vi "Inst_K2002.vi"(8 "error in":errorcluster, 10 "All Message Queues in":T1, 11 "Prueba31 in":refnum<class "Prueba21.lvclass">) -> (0 "error out":errorcluster)   [LabVIEW 2019, in "Prueba21.lvclass"]
uses:
  Prueba21.lvclass
  QMH/Message Queue/All Message Queues.ctl
  QMH/Message Queue/Message Cluster.ctl
  Prueba21.lvclass/Prueba21.ctl
  <vilib>/Utility/error.llb/Error Cluster From Error Code.vi
  QMH/Message Queue/Enqueue Message (Single).vi
  <vilib>/ErrorRing/Error Ring.xnode
  QMH/Message Queue/Message Queue.lvlib
  Instrumento/Keithley2002/Keithley2002.lvclass
panel:
  out "All States":string[](array[string])
  out "Actual State":string
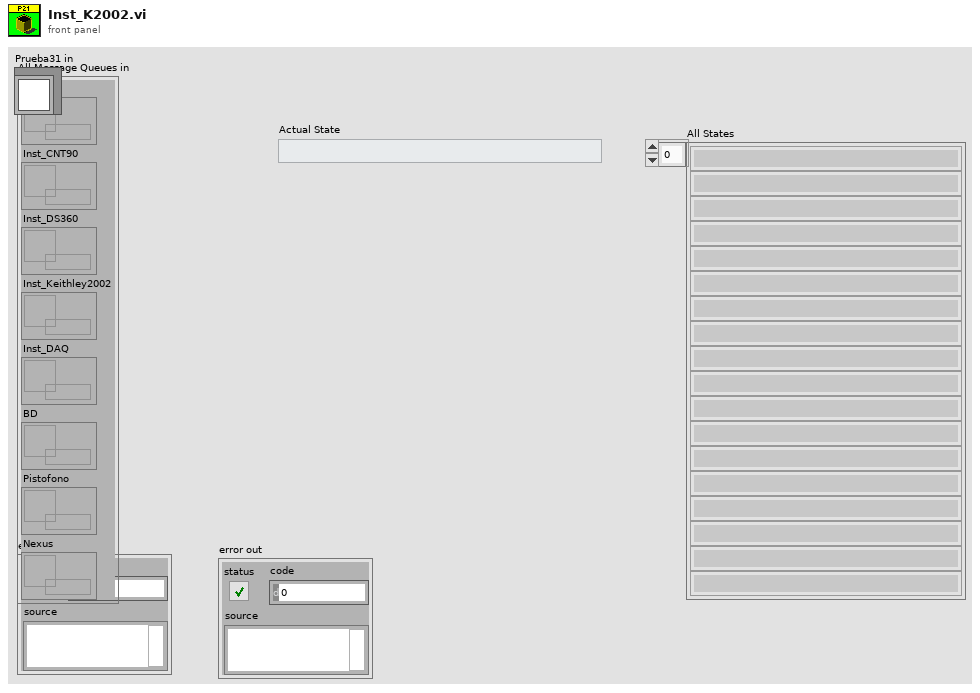
[diagram p1: front panel]
types:
  T1 = typedef "Message Queue.lvlib/All Message Queues.ctl" = cluster{"MHL":refnum<queue>, "Inst_CNT90":refnum<queue>, "Inst_DS360":refnum<queue>, "Inst_Keithley2002":refnum<queue>, "Inst_DAQ":refnum<queue>, "BD":refnum<queue>, "Pistofono":refnum<queue>, "Nexus":refnum<queue>}
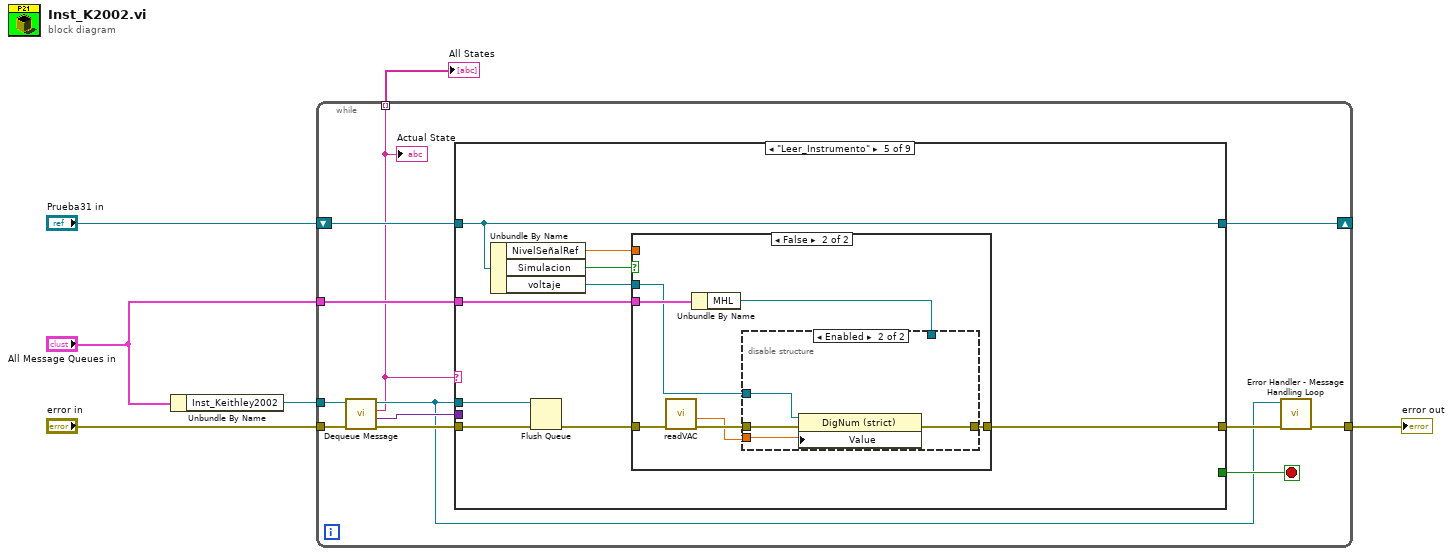
[diagram p0: block diagram]
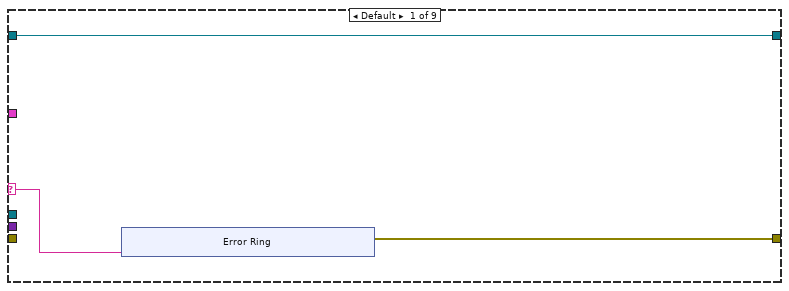
[diagram p2: hidden frame]
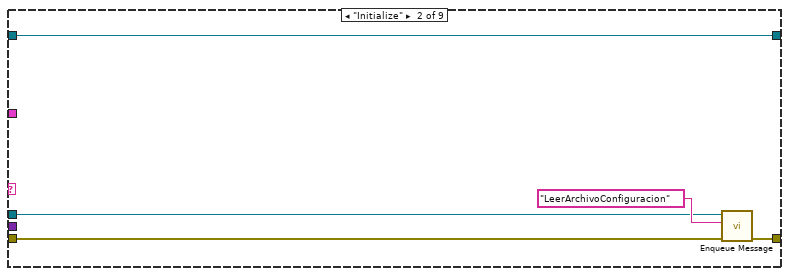
[diagram p3: hidden frame]
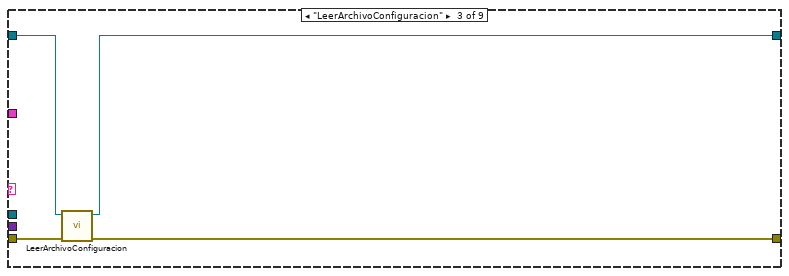
[diagram p4: hidden frame]
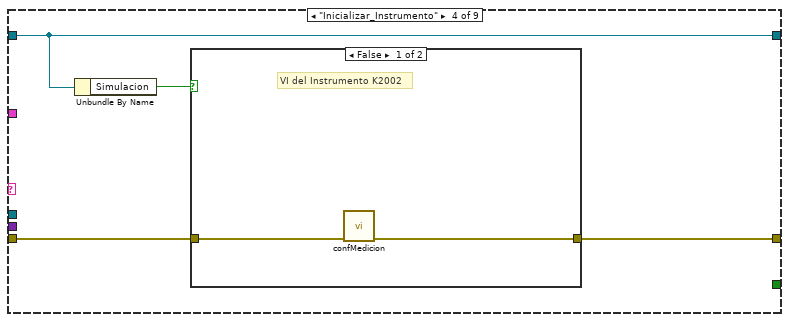
[diagram p5: hidden frame]
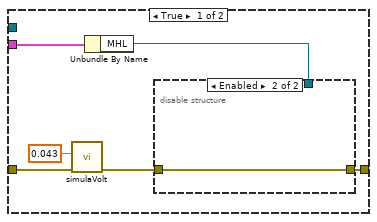
[diagram p7: hidden frame]
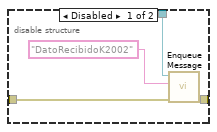
[diagram p8: hidden frame]
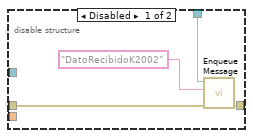
[diagram p9: hidden frame]
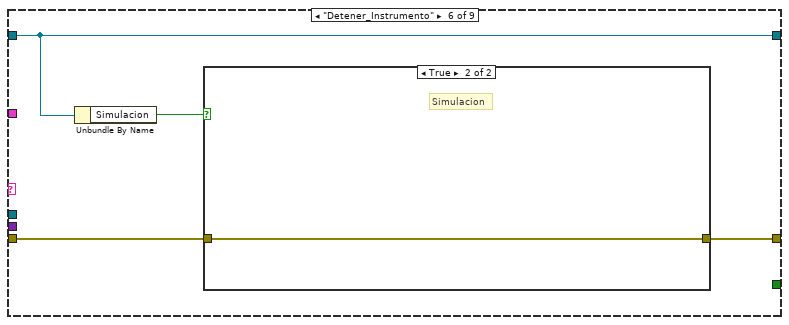
[diagram p10: hidden frame]
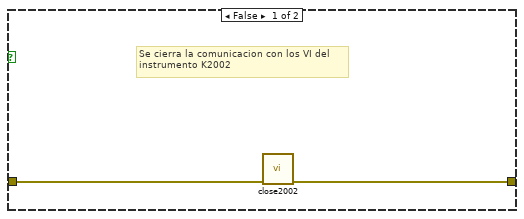
[diagram p11: hidden frame]
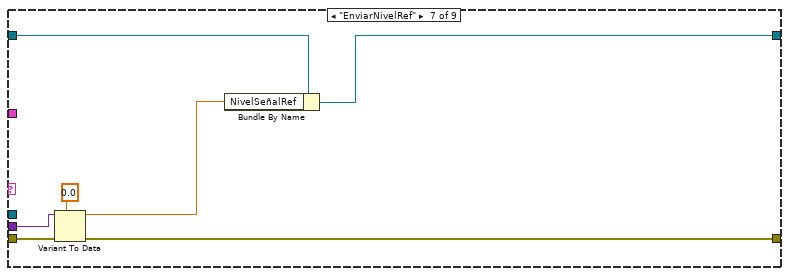
[diagram p12: hidden frame]
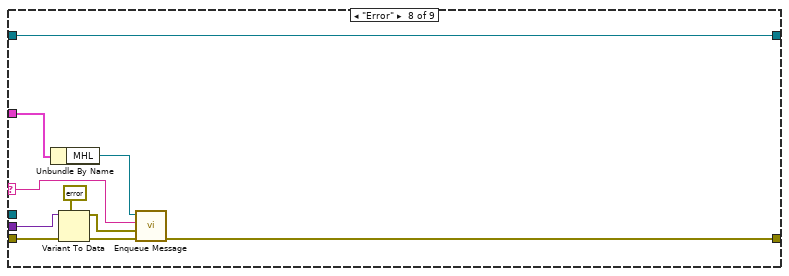
[diagram p13: hidden frame]
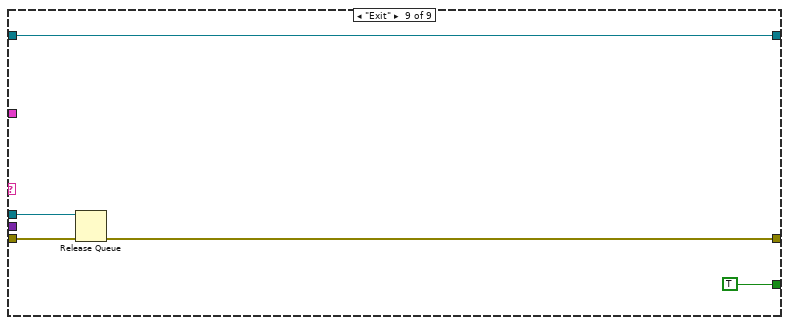
[diagram p14: hidden frame]
diagram:
  n1 = Unbundle By Name("All Message Queues in") -> ("Inst_Keithley2002"=w4:refnum<queue>)
  n2 = while {
    tunnel: "error in" -> [w18]
    tunnel: w4 -> [w17]
    tunnel: "All Message Queues in" -> [w16]
    tunnel: [w9] -> w2
    shift-right: [w12] -> _
    shift-left: "Prueba31 in" -> [w15]
    tunnel: [w7] -> w1 mode=indexing
    stop <- w11 stop-if-true
    n3 = call "Dequeue Message.vi"("error in (no error)"=w18, "Message Queue"=w17) -> ("error out"=w13:errorcluster, "Message Data"=w14:variant, "Message"=w7:string, "dup Message Queue"=w8:refnum<queue>)  [unwired: 6 in]
    "Actual State" <- w7
    n4 = case shown="\"Leer_Instrumento\"" w7 {
      selector: w7 -> [w21 _ _ _ _ _ _ w96 _]
      tunnel: w16 -> [_ _ _ _ w51 _ _ w95 _]
      tunnel: w15 -> [w19 w33 w34 w38 w53 w82 w88 w103 w105]
      tunnel: w8 -> [_ w29 _ _ w47 _ _ _ w107]
      tunnel: w14 -> [_ _ _ _ _ _ w90 w100 _]
      tunnel: w13 -> [_ w31 w36 w39 w50 w80 w92 w101 w108]
      tunnel: [w20 w30 w37 w41 w46 w83 w93 w98 w104] -> w10
      tunnel: [w19 w33 w35 w38 w53 w82 w89 w103 w105] -> w12
      tunnel: [_ _ _ _ _ _ _ _ TRUE] -> w11
      frame Default {
        n5 = xnode "Error Ring"("parameter 0"=w21) -> ("error out"=w20:errorcluster)
      }
      frame "Initialize" {
        n6 = call-poly "Enqueue Message.vi"("error in (no error)"=w31, "Message"="LeerArchivoConfiguracion", "Message Queue"=w29) -> ("error out"=w30:errorcluster)  [unwired: 7 in, 1 out]
      }
      frame "LeerArchivoConfiguracion" {
        n7 = call "LeerArchivoConfiguracion.vi"("error in"=w36, "Prueba31 in"=w34) -> ("error out"=w37:errorcluster, "Prueba31 out"=w35:refnum<class "Prueba21.lvclass">)  [unwired: 8 in]
      }
      frame "Inicializar_Instrumento" {
        n8 = Unbundle By Name(w38) -> ("Simulacion"=w40:bool)
        n9 = case shown="False" w40 {
          tunnel: [w43 w44] -> w41
          tunnel: w39 -> [w42 w44]
          frame False {
            # "VI del Instrumento K2002"
            n10 = call "confMedicion.vi"("error in (no error)"=w42) -> ("error out"=w43:errorcluster)  [unwired: 9 in, 1 out]
          }
          frame True {
            # "Simulacion"
          }
        }
      }
      frame "Leer_Instrumento" {
        n11 = Unbundle By Name(w53) -> ("NivelSeñalRef"=w49:dbl, "Simulacion"=w52:bool, "voltaje"=w45:refnum<vi>)
        n12 = Flush Queue(queue=w47, error in (no error)=w50) -> (error out=w48:errorcluster)  [unwired: 2 out]
        n13 = case shown="False" w52 {
          tunnel: w51 -> [w59 w71]
          tunnel: [w56 w70] -> w46
          tunnel: w48 -> [w58 w68]
          tunnel: w49 -> [_ _]
          tunnel: w45 -> [_ w66]
          frame True {
            n14 = call "simulaVolt.vi"("error in (no error)"=w58, "volt in"=0.043) -> ("error out"=w57:errorcluster)  [unwired: 7 in, 2 out]
            n15 = Unbundle By Name(w59) -> ("MHL"=w55:refnum<queue>)
            n16 = disable-structure shown="Enabled" {
              disable-tunnel: w57 -> [w63 w64]
              disable-tunnel: [w62 w64] -> w56
              disable-tunnel: w55 -> [w61 _]
              frame Disabled {
                n17 = call-poly "Enqueue Message.vi"("error in (no error)"=w63, "Message"="DatoRecibidoK2002", "Message Queue"=w61) -> ("error out"=w62:errorcluster)  [unwired: 7 in, 1 out]
              }
              frame Enabled {
              }
            }
          }
          frame False {
            n18 = call "readVAC.vi"("error in (no error)"=w68) -> ("error out"=w67:errorcluster, "medicion"=w65:dbl)  [unwired: 7 in, 2 out]
            n19 = Unbundle By Name(w71) -> ("MHL"=w69:refnum<queue>)
            n20 = disable-structure shown="Enabled" {
              disable-tunnel: [w75 w78] -> w70
              disable-tunnel: w69 -> [w74 _]
              disable-tunnel: w67 -> [w72 w79]
              disable-tunnel: w66 -> [_ w77]
              disable-tunnel: w65 -> [_ w76]
              frame Disabled {
                n21 = call-poly "Enqueue Message.vi"("error in (no error)"=w72, "Message"="DatoRecibidoK2002", "Message Queue"=w74) -> ("error out"=w75:errorcluster)  [unwired: 7 in, 1 out]
              }
              frame Enabled {
                n22 = property class="DigNum (strict)"(reference=w77, error in=w79, "Value"=w76) -> (error out=w78:errorcluster)  [unwired: 1 out]
              }
            }
          }
        }
      }
      frame "Detener_Instrumento" {
        n23 = Unbundle By Name(w82) -> ("Simulacion"=w81:bool)
        n24 = case shown="True" w81 {
          tunnel: [w85 w86] -> w83
          tunnel: w80 -> [w84 w86]
          frame False {
            # "Se cierra la comunicacion con los VI del\ninstrumento K2002"
            n25 = call "close2002.vi"("error in (no error)"=w84) -> ("error out"=w85:errorcluster)  [unwired: 9 in, 1 out]
          }
          frame True {
            # "Simulacion"
          }
        }
      }
      frame "EnviarNivelRef" {
        n26 = Variant To Data(error in=w92, type=0.0, Variant=w90) -> (data=w87:dbl, error out=w93:errorcluster)
        n27 = Bundle By Name(cluster=w88, "NivelSeñalRef"=w87) -> (w89:refnum<class "Prueba21.lvclass">)
      }
      frame "Error" {
        n28 = Unbundle By Name(w95) -> ("MHL"=w94:refnum<queue>)
        n29 = Variant To Data(error in=w101, type=errorcluster {"status"=FALSE, "code"=0, "source"=""} ("error constant"), Variant=w100) -> (data=w97:errorcluster, error out=w99:errorcluster)
        n30 = call-poly "Enqueue Message.vi"("error in (no error)"=w99, "Message Data"=w97, "Message"=w96, "Message Queue"=w94) -> ("error out"=w98:errorcluster)  [unwired: 6 in, 1 out]
      }
      frame "Exit" {
        n31 = Release Queue(queue=w107, error in (no error)=w108) -> (error out=w104:errorcluster)  [unwired: 1 in, 2 out]
      }
    }
    n32 = call "Error Handler - Message Handling Loop.vi"("error in (no error)"=w10, "Message Queue"=w8) -> ("dup error in"=w9:errorcluster)  [unwired: 8 in, 1 out]
  }
  "error out" <- w2
  "All States" <- w1
